vi "Read Temperature Covesion.vi"() -> ()   [LabVIEW 2009]
panel:
  out "error out":errorcluster
  out "Temperature":dbl=47.423
  in  "error in (no error)":errorcluster
  in  "VISA resource name":refnum<visa-resource-name>="COM6"
  # "V1.02"
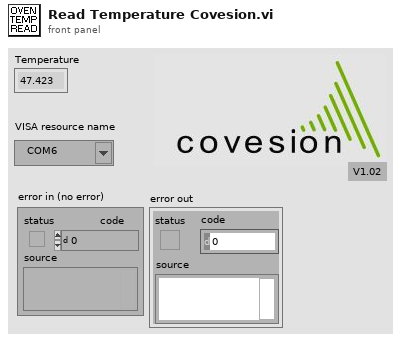
[diagram p1: front panel]
types:
  T1 = cluster{"Setpoint":dbl, "Temperature":dbl, "Control":i32, "Output %":dbl, "Alarms":i32, "Faults":i32, "TEMP OK":i32, "Supply VDC":dbl, "Version":dbl, "Test cycle":i32, "Test Mode":i32, "Checksum":i32}
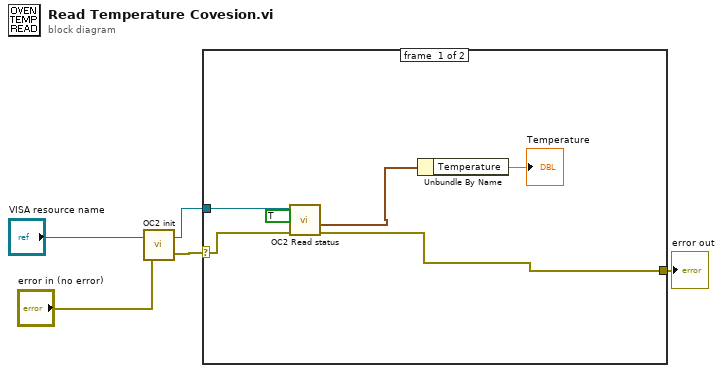
[diagram p0: block diagram]
diagram:
  n1 = call "OC2 init.vi"("error in (no error)"="error in (no error)", "VISA resource name"="VISA resource name") -> ("error out"=w2:errorcluster, "duplicate VISA resource name"=w3:refnum<visa-resource-name>)
  n2 = case shown="No Error" w2 {
    selector: w2 -> [w7 w12]
    tunnel: w3 -> [w11 _]
    tunnel: [w6 w12] -> w1
    frame #0 {
      n3 = call "OC2 Read status.vi"("VISA resource name"=w11, "enable"=TRUE, "error in"=w7) -> ("Report cluster"=w9:T1, "error out"=w6:errorcluster)  [unwired: 1 in, 3 out]
      n4 = Unbundle By Name(w9) -> ("Temperature"=→"Temperature":dbl)
    }
    frame #1 {
    }
  }
  "error out" <- w1
